vi "Drawboard.vi"(1 "Board":i32[][](array[numeric])) -> (0 "2D Picture":picture)   [LabVIEW 2025]
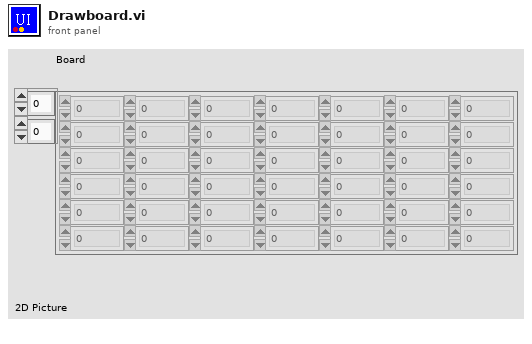
[diagram p1: front panel]
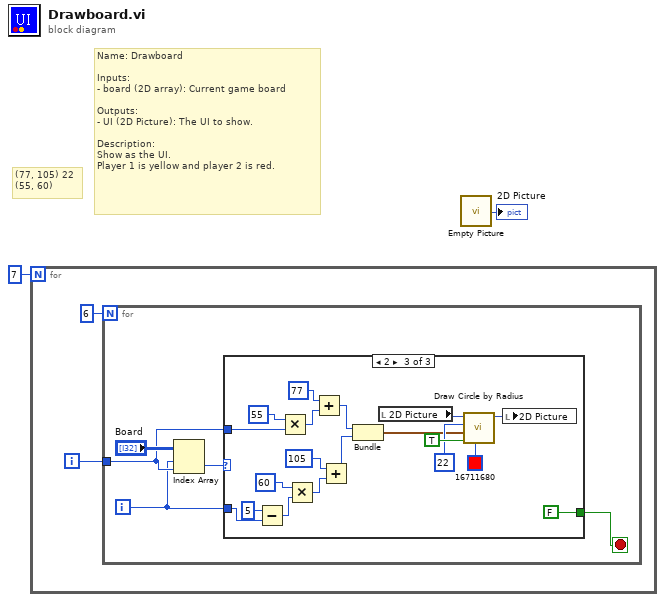
[diagram p0: block diagram]
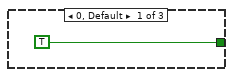
[diagram p2: hidden frame]
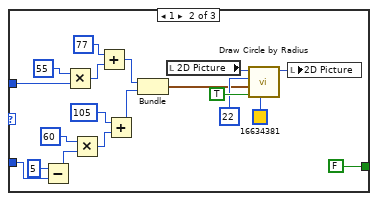
[diagram p3: hidden frame]
diagram:
  # "Name: Drawboard\n\nInputs:\n- board (2D array): Current game board\n\nOutputs:\n- UI (2D Picture): The UI to show.\n\nDescription:\nShow as the UI.\nPlayer 1 is yellow and player 2 is red."
  # "(77, 105) 22\n(55, 60)"
  n1 = for {
    N: 7 -> [_]
    i -> [w3]
    n2 = for {
      N: 6 -> [_]
      tunnel: w3 -> [w6]
      i -> [w5]
      stop <- w7 stop-if-true
      n3 = Index Array(array="Board", index (row)=w5, index (col)=w6) -> (element=w8:i32)
      n4 = case shown="2" w8 {
        tunnel: [TRUE FALSE FALSE] -> w7
        tunnel: w6 -> [_ w27 w46]
        tunnel: w5 -> [_ w11 w32]
        frame 0, Default {
        }
        frame 1 {
          n5 = Subtract(x=5, y=w11) -> (x-y=w12:i32)
          n6 = Multiply(x=55, y=w27) -> (x*y=w25:i32)
          n7 = Multiply(x=60, y=w12) -> (x*y=w24:i32)
          n8 = Add(x=77, y=w25) -> (x+y=w21:i32)
          n9 = Add(x=105, y=w24) -> (x+y=w20:i32)
          n10 = Bundle(w21, w20) -> (w17:cluster{i32, i32})  [unwired: 1 in]
          n11 = local read "2D Picture"() -> (w14:picture)
          n12 = call <vilib>:"Draw Circle by Radius.vi"("color(black)"=u32 16634381, "fill?(F)"=TRUE, "pixel center"=w17, "radius"=i16 22, "picture"=w14) -> ("new picture"=w15:picture)  [unwired: 6 in]
          n13 = local write "2D Picture"(w15) -> ()
        }
        frame 2 {
          n14 = Subtract(x=5, y=w32) -> (x-y=w30:i32)
          n15 = Multiply(x=55, y=w46) -> (x*y=w44:i32)
          n16 = Multiply(x=60, y=w30) -> (x*y=w43:i32)
          n17 = Add(x=77, y=w44) -> (x+y=w41:i32)
          n18 = Add(x=105, y=w43) -> (x+y=w40:i32)
          n19 = Bundle(w41, w40) -> (w37:cluster{i32, i32})  [unwired: 1 in]
          n20 = local read "2D Picture"() -> (w34:picture)
          n21 = call <vilib>:"Draw Circle by Radius.vi"("color(black)"=u32 16711680, "fill?(F)"=TRUE, "pixel center"=w37, "radius"=i16 22, "picture"=w34) -> ("new picture"=w35:picture)  [unwired: 6 in]
          n22 = local write "2D Picture"(w35) -> ()
        }
      }
    }
  }
  n23 = call "Empty Picture"() -> ("empty picture"=→"2D Picture":picture)
